vi "AcquisitionDiagram.vi"() -> ()   [LabVIEW 2017]
panel:
  in  "empty picture":picture
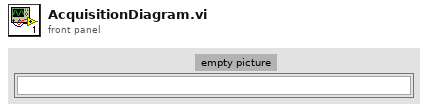
[diagram p1: front panel]
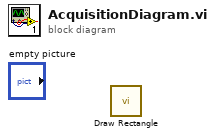
[diagram p0: block diagram]
diagram:
  n1 = call <vilib>:"Draw Rectangle.vi"() -> ()  [unwired: 9 in, 1 out]
